vi "Cmd getData.vi"(4 "error in (no error)":errorcluster, 7 "command reference":T3) -> (0 "error out":errorcluster, 1 "object is locked?":bool, 2 "data":T1, 3 "command reference out":T3)   [LabVIEW 2012, in "NI_Database_API_64.lvlib"]
doc: "Returns the data of a <B>Command</B> object.\n\nIf the object is currently locked for modification, <B>object is locked?</B> will return TRUE.\n\n[GOOP 1.0/1.0]"
uses:
  NI_Database_API_64.lvlib
  Cmd DataMembers.ctl
  Connection.llb/Conn ObjectReference.ctl
  Cmd ObjectReference.ctl
  <vilib>/Utility/_goopsup.llb/GOOP Object Repository Method.ctl
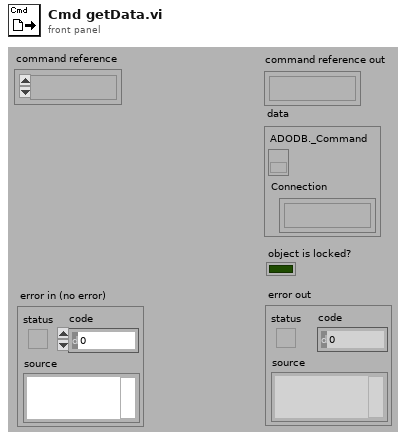
[diagram p1: front panel]
types:
  T1 = typedef "NI_Database_API_64.lvlib/Cmd DataMembers.ctl" = cluster{"ADODB._Command":refnum<k7>, "Connection":T2}
  T2 = typedef "NI_Database_API_64.lvlib/Conn ObjectReference.ctl" = refnum<k1>
  T3 = typedef "NI_Database_API_64.lvlib/Cmd ObjectReference.ctl" = refnum<k1>
  T4 = typedef "GOOP Object Repository Method.ctl" = enum16{"Create", "GetCopy", "GetModify", "Set", "Destroy", "Create Static", "Get All Refs", "Reset", "Get Statistics"}
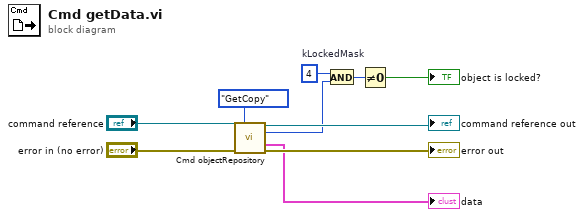
[diagram p0: block diagram]
diagram:
  w2 = 4  # kLockedMask
  n1 = call "Cmd objectRepository.vi"("command reference"="command reference", "method"=GOOP_Object_Repository_Method."GetCopy", "error in (no error)"="error in (no error)") -> ("command reference out"=→"command reference out":T3, "flags out"=w1:i32, "classDataOut"=→"data":T1, "error out"=→"error out":errorcluster)  [unwired: 6 in, 3 out]
  n2 = And(x=w2, y=w1) -> (x .and. y?=w3:i32)
  n3 = Not Equal To 0?(x=w3) -> (x != 0?=→"object is locked?":bool)
